vi "Tear Down.vi"(8 "error in (no error)":errorcluster, 11 "Replay in":refnum<class "Replay.lvclass">) -> (0 "error out":errorcluster, 3 "Replay out":refnum<class "Replay.lvclass">)   [LabVIEW 2016, in "CLD Exam - ATM.lvlib" / "Replay.lvclass"]
uses:
  Replay.lvclass
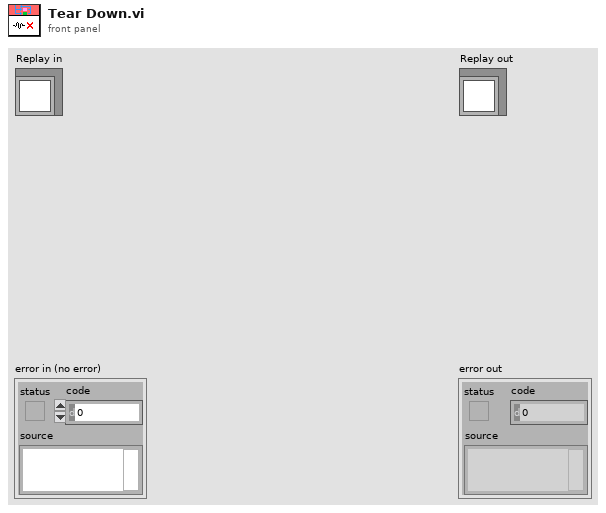
[diagram p1: front panel]
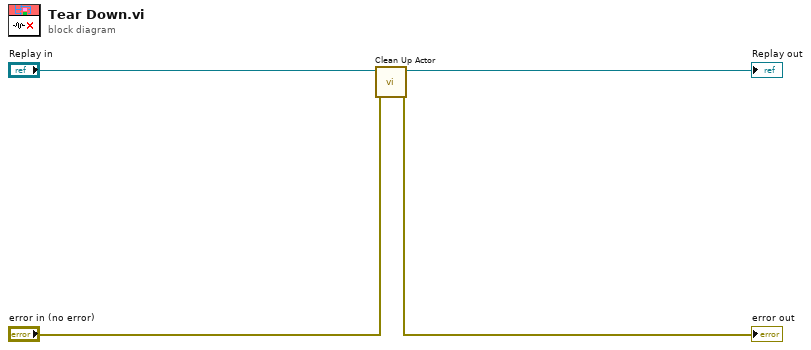
[diagram p0: block diagram]
diagram:
  n1 = call-dynamic "Clean Up Actor.vi"("error in (no error)"="error in (no error)", "Replay in"="Replay in") -> ("error out"=→"error out":errorcluster, "Replay out"=→"Replay out":refnum<class "Replay.lvclass">)  [unwired: 8 in]
